vi "Fire DAQMeasSettingsChanged Event_DAQ.vi"(8 "error in (no error)":errorcluster, 9 "vData":variant, 10 "Measurement config":T1={"Data Rate 9775"=3.0, "Data Rate 9215"=1200000.0, "Samples RMS 9215"=480000, "Samples RMS 9775"=3}, 11 "DAQ_Engine in":refnum<class "DAQ_Engine.lvclass">) -> (0 "error out":errorcluster, 3 "DAQ_Engine out":refnum<class "DAQ_Engine.lvclass">)   [LabVIEW 2019, in "DAQ_Engine.lvclass"]
doc: "Developed by Kevin Thompson\nkevin@thompsonengineering.net\n\nCopyright 2018-2020\nThompson Engineering, LLC"
uses:
  DAQ_Engine.lvclass
  Common/DataTypes/Measurement Config--cluster.ctl
  DataTypes/DAQMeasSettingsChg EvData--cluster.ctl
  DataTypes/DAQMeasSettingsEvData--cluster.ctl
  DAQ_Engine.lvclass/DAQ_Engine.ctl
  Accessors/Get PublicEvents.vi
  Accessors/Get MeasSettings.vi
  Accessors/Set MeasSettings.vi
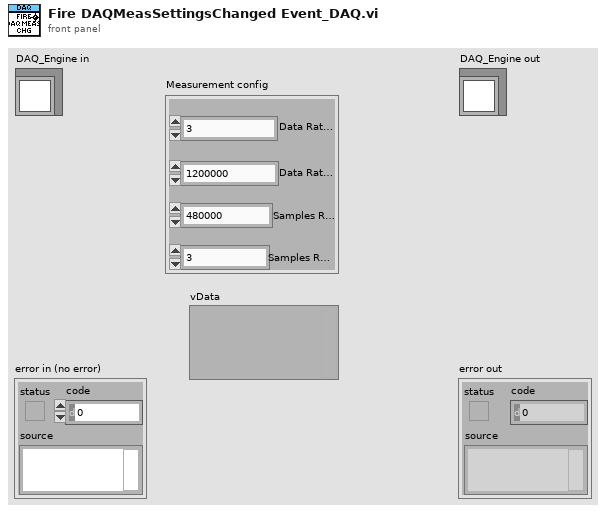
[diagram p1: front panel]
types:
  T1 = typedef "Measurement Config--cluster.ctl" = cluster{"Data Rate 9775":dbl, "Data Rate 9215":dbl, "Samples RMS 9215":u32, "Samples RMS 9775":u32}
  T2 = typedef "DAQ_Engine.lvclass/DAQMeasSettingsChg EvData--cluster.ctl" = cluster{"Time Stamp":timestamp, "OLD Settings":T3, "NEW Settings":T3}
  T3 = typedef "DAQ_Engine.lvclass/DAQMeasSettingsEvData--cluster.ctl" = cluster{"Measurement config":T1, "vData":variant}
  T4 = typedef "DAQ_Engine.lvclass/Public Events--cluster.ctl" = cluster{"DAQ_Engine.AsyncCmd Event":refnum<user-event>, "DAQ_Engine.AsyncMsg Event":refnum<user-event>, "stop process":refnum<user-event>, "DAQ_Engine.DAQStateChg Ev":refnum<user-event>, "DAQ_Engine.MeasSettingsChg Ev":refnum<user-event>, "DAQ_Engine.AcqModeChg Ev":refnum<user-event>}
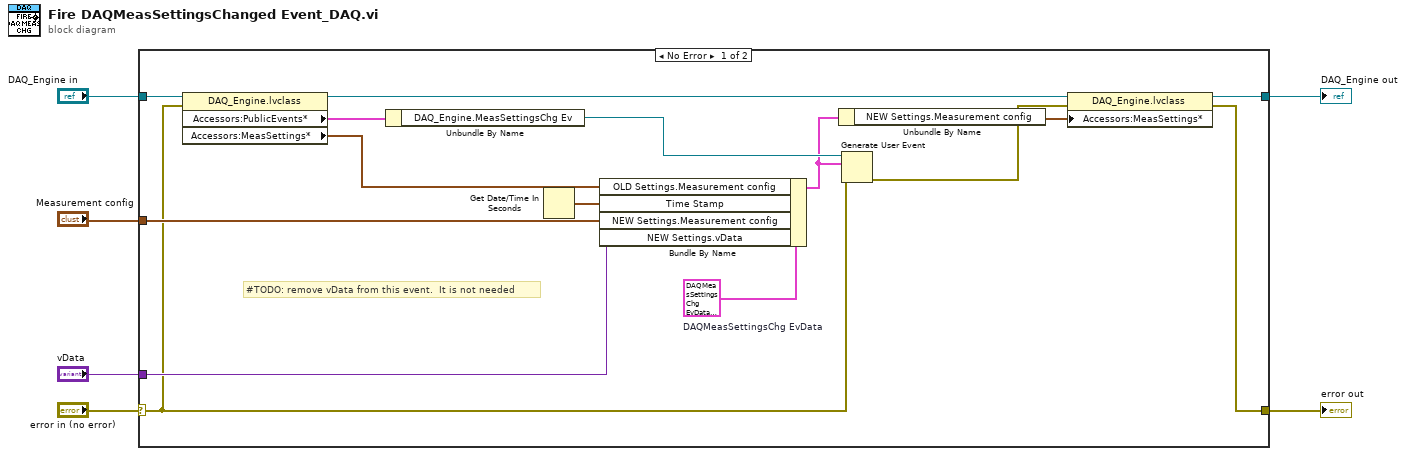
[diagram p0: block diagram]
diagram:
  n1 = case shown="No Error" "error in (no error)" {
    selector: "error in (no error)" -> [w8 w23]
    tunnel: [w15 w23] -> w5
    tunnel: [w18 w22] -> w3
    tunnel: "DAQ_Engine in" -> [w20 w22]
    tunnel: "Measurement config" -> [w9 _]
    tunnel: "vData" -> [w19 _]
    frame No Error {
      w10 = T2 {"Time Stamp"=timestamp(0 s since 1904-01-01), "OLD Settings"={"Measurement config"={"Data Rate 9775"=3.0, "Data Rate 9215"=1200000.0, "Samples RMS 9215"=480000, "Samples RMS 9775"=3}, "vData"=variant}, "NEW Settings"={"Measurement config"={"Data Rate 9775"=3.0, "Data Rate 9215"=1200000.0, "Samples RMS 9215"=480000, "Samples RMS 9775"=3}, "vData"=variant}}  # DAQMeasSettingsChg EvData
      # "#TODO: remove vData from this event.  It is not needed"
      n2 = property class="DAQ_Engine.lvclass"(reference=w20, error in=w8) -> (reference out=w11:refnum<class "DAQ_Engine.lvclass">, "Accessors:PublicEvents*"=w12:T4, "Accessors:MeasSettings*"=w13:T1)  [unwired: 1 out]
      n3 = Unbundle By Name(w12) -> ("DAQ_Engine.MeasSettingsChg Ev"=w14:refnum<user-event>)
      n4 = Get Date/Time In Seconds() -> (seconds since 1Jan1904=w21:timestamp)
      n5 = Bundle By Name(cluster=w10, "OLD Settings.Measurement config"=w13, "Time Stamp"=w21, "NEW Settings.Measurement config"=w9, "NEW Settings.vData"=w19) -> (w7:T2)
      n6 = Unbundle By Name(w7) -> ("NEW Settings.Measurement config"=w17:T1)
      n7 = Generate User Event(user event=w14, event data cluster=w7, error in=w8) -> (error out=w16:errorcluster)  [unwired: 1 in, 1 out]
      n8 = property class="DAQ_Engine.lvclass"(reference=w11, error in=w16, "Accessors:MeasSettings*"=w17) -> (reference out=w18:refnum<class "DAQ_Engine.lvclass">, error out=w15:errorcluster)
    }
    frame Error {
    }
  }
  "error out" <- w5
  "DAQ_Engine out" <- w3
